vi "pulse_generator_multiheater_partial_refnum.vi"(2 "Stop! Refnum":refnum<vi>, 3 "Pulse Generator Control Multiheater Refnums":T1) -> ()   [LabVIEW 2017]
uses:
  pulse_generator_controls_multiheater_refnums.ctl
  <vilib>/Utility/error.llb/DialogType.ctl
  <vilib>/DAQmx/write.llb/DAQmx Write (Digital 1D Bool NChan 1Samp 1Line).vi
  <vilib>/DAQmx/write.llb/DAQmx Write (Digital Wfm 1Chan NSamp).vi
  <vilib>/DAQmx/write.llb/DAQmx Write (Counter 1D Frequency 1Chan NSamp).vi
  <vilib>/DAQmx/read.llb/DAQmx Read (Counter DBL 1Chan 1Samp).vi
  <vilib>/DAQmx/create/channels.llb/DAQmx Create Channel (CI-Position-Angular Encoder).vi
  <vilib>/DAQmx/create/channels.llb/DAQmx Create Channel (DO-Digital Output).vi
  <vilib>/DAQmx/configure/timing.llb/DAQmx Timing (Sample Clock).vi
  <vilib>/DAQmx/create/channels.llb/DAQmx Create Channel (CO-Pulse Generation-Frequency).vi
  <vilib>/DAQmx/configure/timing.llb/DAQmx Timing (Implicit).vi
  <vilib>/DAQmx/configure/trigger.llb/DAQmx Start Trigger (Digital Edge).vi
  <vilib>/Waveform/DWDTOps.llb/DWDT Uncompress Digital.vi
  <vilib>/DAQmx/miscellaneous.llb/DAQmx Fill In Error Info.vi
panel:
  out "data":dbl format="%0.2f"
  out "Stopped!":bool caption="OK"
  in  "Stop! Local":bool
  out "message":string=" INSTRUCTIONS:\r\rNormal Use:  When using subVIs that incorporate the error in/error out (or error I/O) structure, place this handler where you want to inform the user of an error, typically at the end of the I/O data path, as the last action of the program.  If the error in error? is ERROR, the handler creates a message describing the error and its source.  If the type of dialog = 1 (default), the message is displayed to the user, who can only acknowedge it.  If the type = 2, the user can acknowledge the message or abort execution; aborting a program with active I/O is not recommended.  If the type = 0, no message is displayed; this is used to process the error programmatically, and the error out cluster elements are wired to individual terminals for that reason.  \r\rOther Use:\n\r\nlocal testing.  To test the error code of a subVI or function that does not have the error I/O structure, you can wire its error code and a source string to the local error code and error source inputs.  If error in error? indicates no error and error code is not equal to 0, the local code and source are substituted for the error in values, and error? is set TRUE (ERROR)."
  in  "SwitchHelper":bool
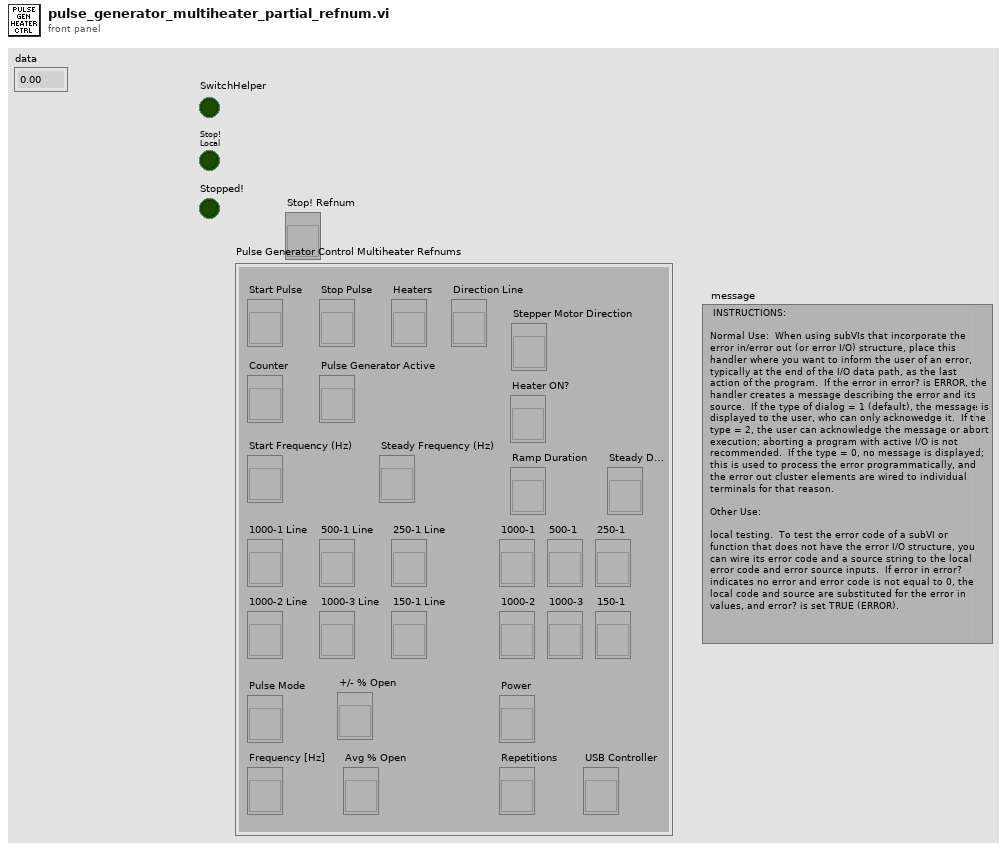
[diagram p1: front panel]
types:
  T1 = typedef "pulse_generator_controls_multiheater_refnums.ctl" = cluster{"Start Pulse":refnum<vi>, "Stop Pulse":refnum<vi>, "Heaters":refnum<vi>, "Counter":refnum<vi>, "Start Frequency (Hz)":refnum<vi>, "Pulse Generator Active":refnum<vi>, "Stepper Motor Direction":refnum<vi>, "Ramp Duration":refnum<vi>, "Direction Line":refnum<vi>, "1000-1 Line":refnum<vi>, "1000-2 Line":refnum<vi>, "1000-3 Line":refnum<vi>, "500-1 Line":refnum<vi>, "250-1 Line":refnum<vi>, "1000-1":refnum<vi>, "1000-2":refnum<vi>, "1000-3":refnum<vi>, "500-1":refnum<vi>, "250-1":refnum<vi>, "150-1":refnum<vi>, "Heater ON?":refnum<vi>, "150-1 Line":refnum<vi>, "Power":refnum<vi>, "Steady Frequency (Hz)":refnum<vi>, "Steady Duration ":refnum<vi>, "Pulse Mode":refnum<vi>, "Frequency [Hz]":refnum<vi>, "Avg % Open":refnum<vi>, "Repetitions":refnum<vi>, "+/- % Open":refnum<vi>, "USB Controller":refnum<vi>}
  T2 = enum8{"Enabled", "Disabled", "Disabled and Grayed Out"}
  T3 = typedef "DialogType.ctl" = u16
  T4 = cluster{"1000-1":refnum<vi>, "1000-2":refnum<vi>, "1000-3":refnum<vi>, "500-1":refnum<vi>, "250-1":refnum<vi>, "150-1":refnum<vi>}
  T5 = cluster{"1000-1 Line":refnum<vi>, "1000-2 Line":refnum<vi>, "1000-3 Line":refnum<vi>, "500-1 Line":refnum<vi>, "250-1 Line":refnum<vi>, "150-1 Line":refnum<vi>}
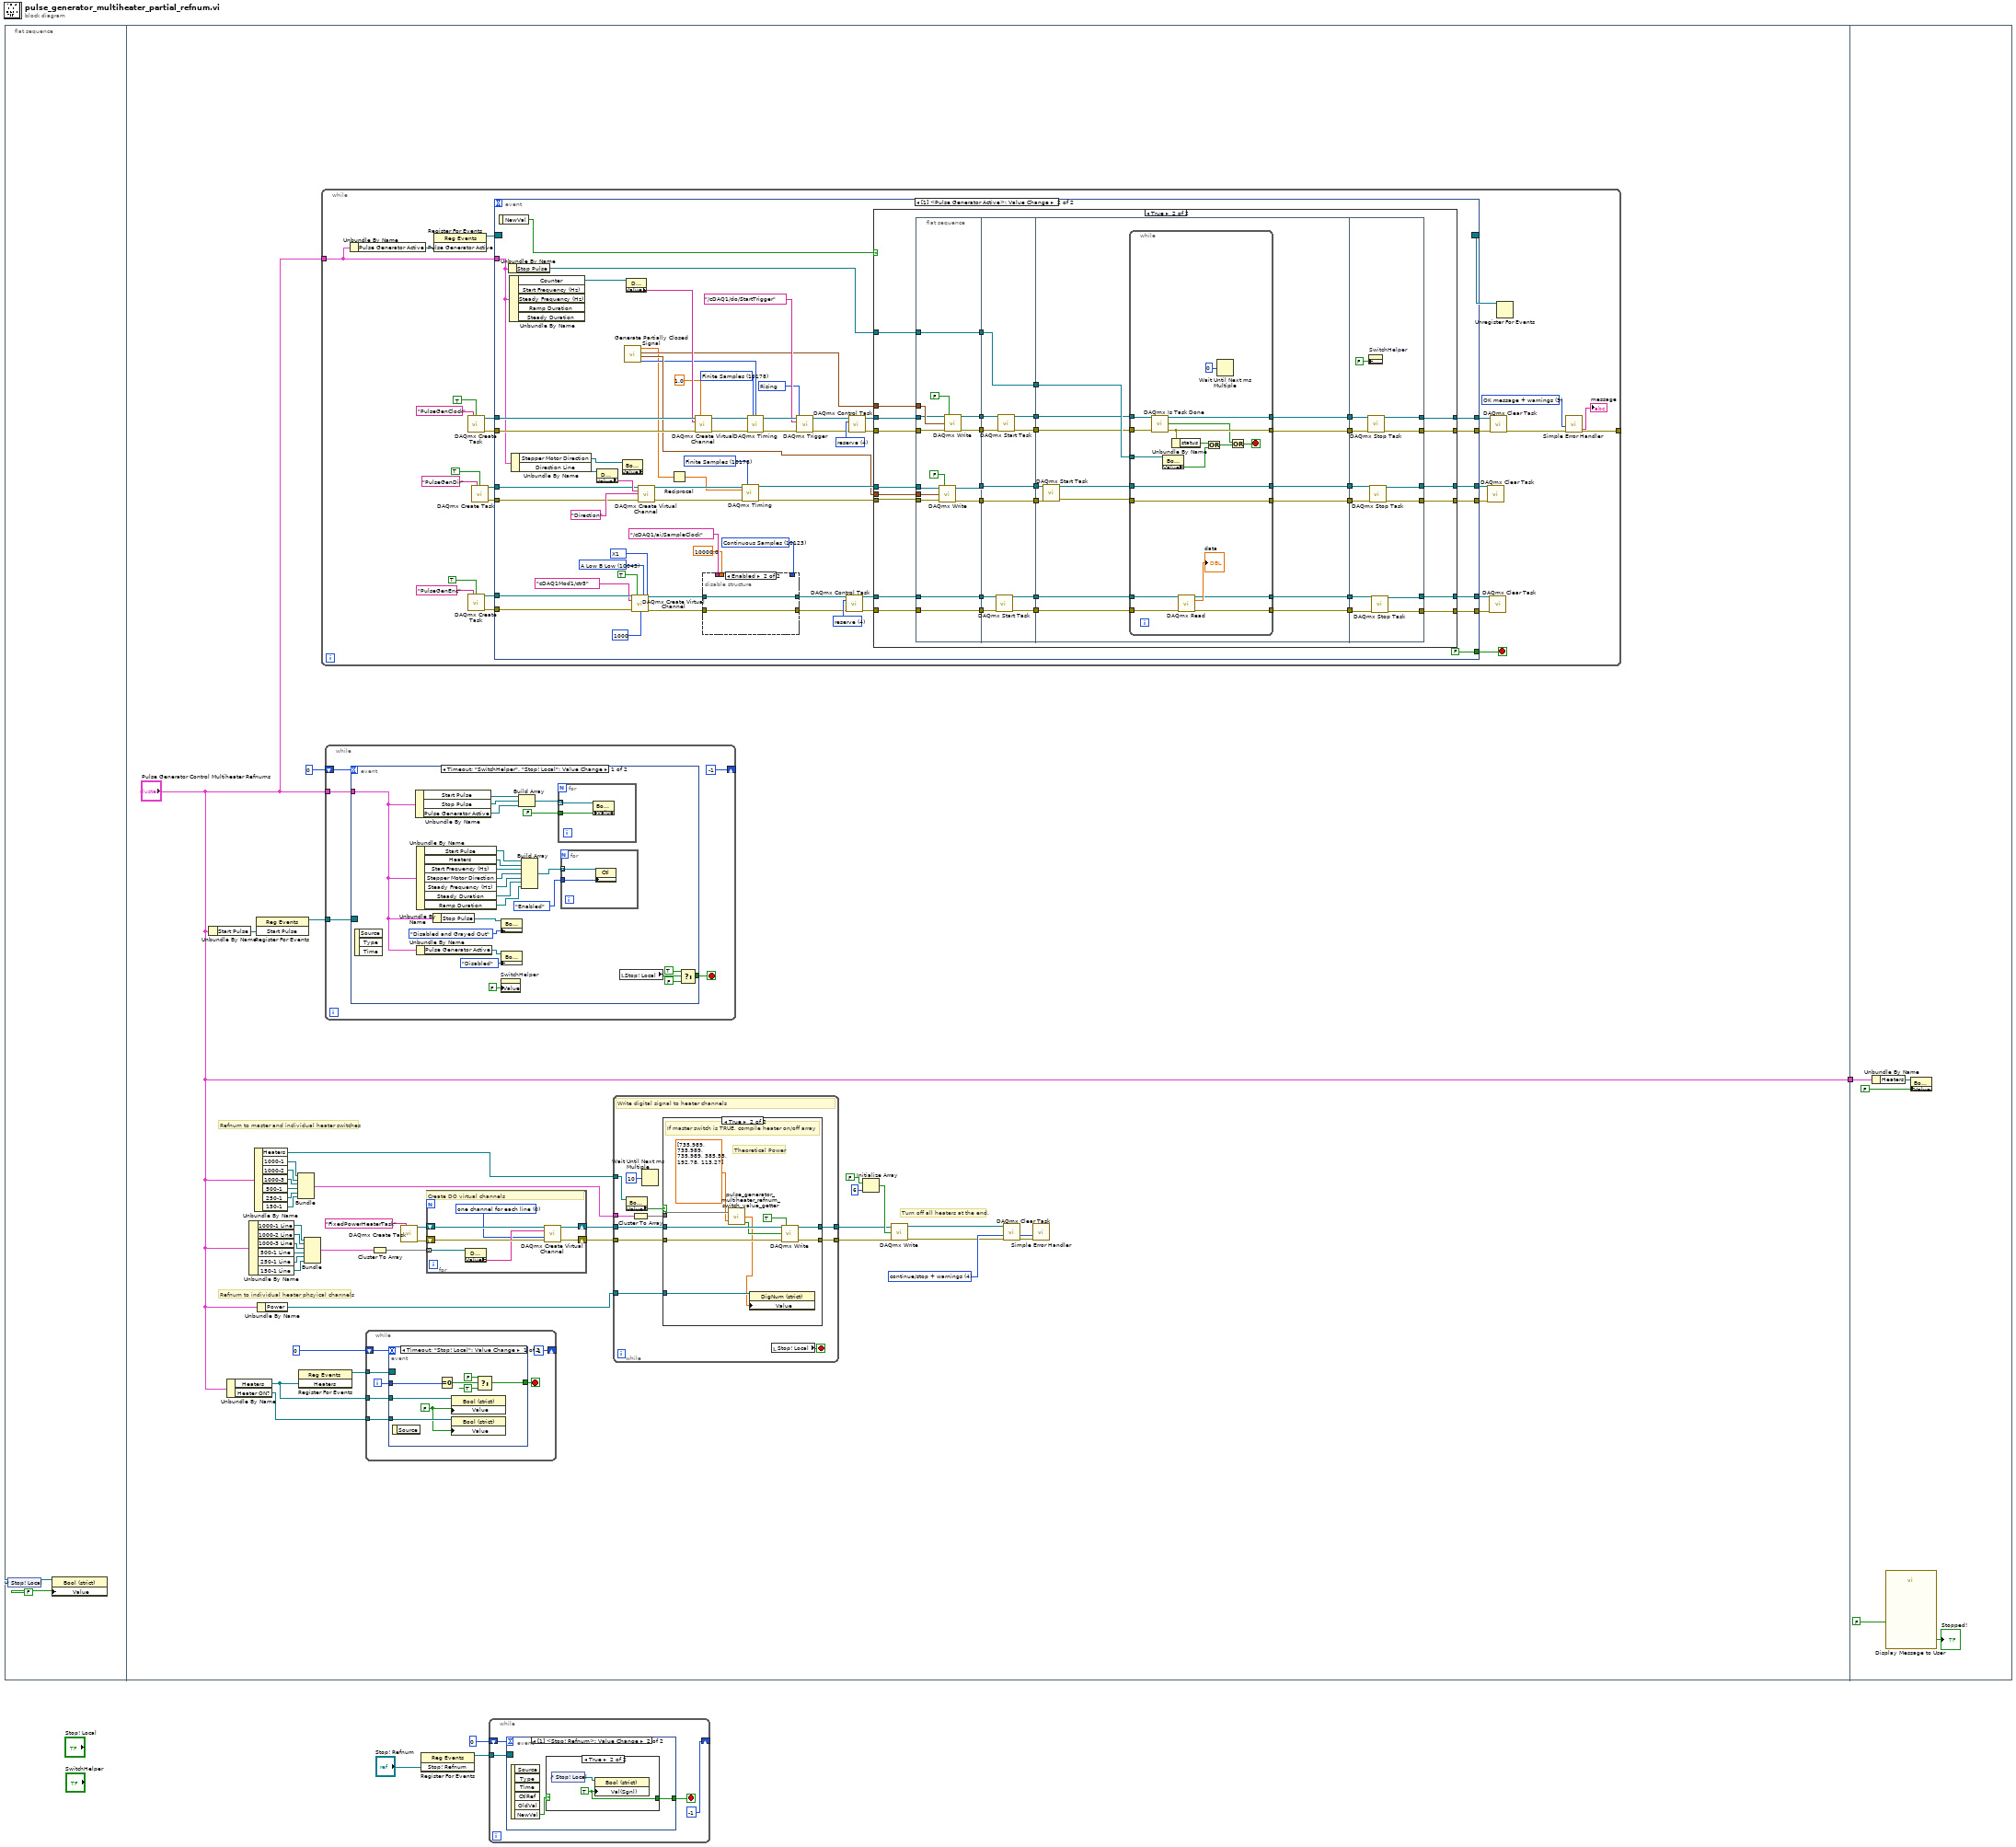
[diagram p0: block diagram]
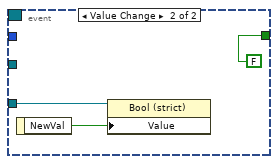
[diagram p2: hidden frame]
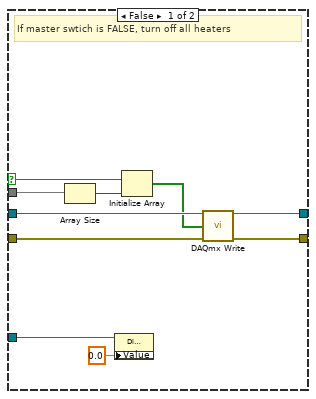
[diagram p3: hidden frame]
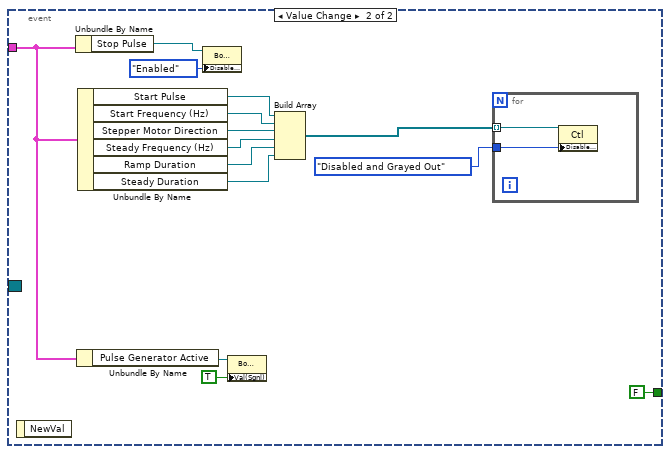
[diagram p4: hidden frame]
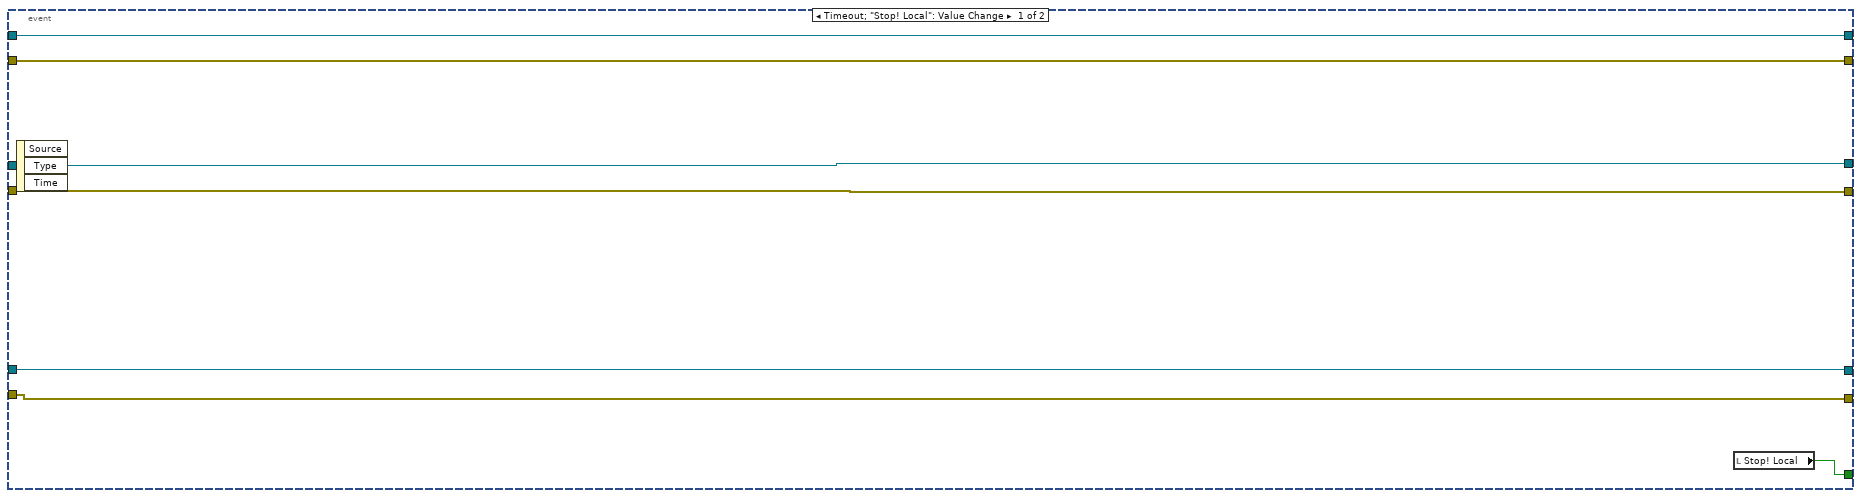
[diagram p5: hidden frame]
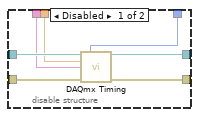
[diagram p6: hidden frame]
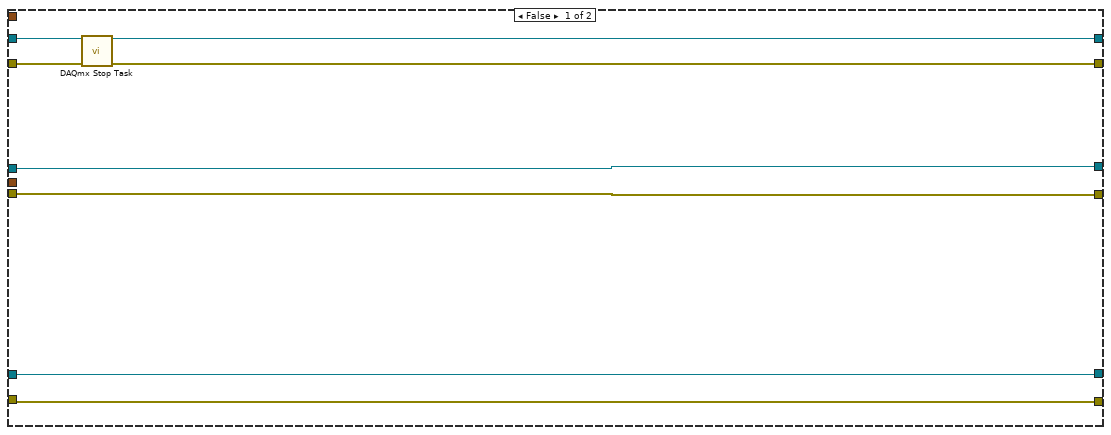
[diagram p7: hidden frame]
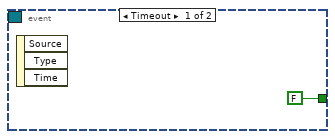
[diagram p8: hidden frame]
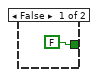
[diagram p9: hidden frame]
diagram:
  n1 = flat-sequence {
    tunnel: ["Pulse Generator Control Multiheater Refnums"] -> w1
    tunnel: w1 -> [w371]
    frame #0 {
      n2 = control-ref of="Stop! Local"() -> (w5:refnum<vi>)
      n3 = property class="Bool (strict)"(reference=w5, "Value"=FALSE) -> ()  [unwired: 1 in, 2 out]
    }
    frame #1 {
      w40 = T3 4 items=["no dialog", "OK message", "continue or stop message", "OK message + warnings", "continue/stop + warnings"] ("type of dialog (OK msg:1)")
      # "Turn off all heaters at the end."
      # "Refnum to individual heater phsyical channels"
      # "Refnum to master and individual heater switches"
      n4 = Unbundle By Name("Pulse Generator Control Multiheater Refnums") -> ("Start Pulse"=w43:refnum<vi>)
      n5 = Unbundle By Name("Pulse Generator Control Multiheater Refnums") -> ("Heaters"=w35:refnum<vi>, "Heater ON?"=w17:refnum<vi>)
      n6 = Unbundle By Name("Pulse Generator Control Multiheater Refnums") -> ("1000-1 Line"=w14:refnum<vi>, "1000-2 Line"=w13:refnum<vi>, "1000-3 Line"=w12:refnum<vi>, "500-1 Line"=w11:refnum<vi>, "250-1 Line"=w10:refnum<vi>, "150-1 Line"=w9:refnum<vi>)
      n7 = Unbundle By Name("Pulse Generator Control Multiheater Refnums") -> ("Heaters"=w34:refnum<vi>, "1000-1"=w33:refnum<vi>, "1000-2"=w32:refnum<vi>, "1000-3"=w31:refnum<vi>, "500-1"=w30:refnum<vi>, "250-1"=w28:refnum<vi>, "150-1"=w18:refnum<vi>)
      n8 = register-events(w43) -> (reference out=w44:refnum<event-registration>)  [unwired: 2 in, 1 out]
      n9 = Unbundle By Name("Pulse Generator Control Multiheater Refnums") -> ("Power"=w7:refnum<vi>)
      n10 = Bundle("1000-1"=w33, "1000-2"=w32, "1000-3"=w31, "500-1"=w30, "250-1"=w28, "150-1"=w18) -> (w15:T4)  [unwired: 1 in]
      n11 = register-events(w35) -> (reference out=w39:refnum<event-registration>)  [unwired: 2 in, 1 out]
      n12 = Bundle("1000-1 Line"=w14, "1000-2 Line"=w13, "1000-3 Line"=w12, "500-1 Line"=w11, "250-1 Line"=w10, "150-1 Line"=w9) -> (w16:T5)  [unwired: 1 in]
      n13 = while {
        tunnel: [w162] -> _
        tunnel: "Pulse Generator Control Multiheater Refnums" -> [w161]
        stop <- w170 stop-if-true
        w173 = T3 3 items=["no dialog", "OK message", "continue or stop message", "OK message + warnings", "continue/stop + warnings"] ("type of dialog (OK msg:1)")
        n14 = Unbundle By Name(w161) -> ("Pulse Generator Active"=w163:refnum<vi>)
        n15 = register-events(w163) -> (reference out=w175:refnum<event-registration>)  [unwired: 2 in, 1 out]
        n16 = call <vilib>:"DAQmx Create Task.vi"("new task name"="PulseGenClock", "auto cleanup"=TRUE) -> ("task out"=w172:refnum<k21>, "error out"=w171:errorcluster)  [unwired: 12 in]
        n17 = call <vilib>:"DAQmx Create Task.vi"("new task name"="PulseGenEnc", "auto cleanup"=TRUE) -> ("task out"=w154:refnum<k21>, "error out"=w153:errorcluster)  [unwired: 12 in]
        n18 = call <vilib>:"DAQmx Create Task.vi"("new task name"="PulseGenDir", "auto cleanup"=TRUE) -> ("task out"=w168:refnum<k21>, "error out"=w167:errorcluster)  [unwired: 12 in]
        n19 = event shown="[1] <Pulse Generator Active>: Value Change" {
          selector: w175 -> [_ _]
          dyn-events: [_ _] -> w160
          timeout: _ -> [_ _]
          tunnel: [w183 w224] -> w177
          tunnel: [w184 w223] -> w176
          tunnel: w172 -> [w184 w242]
          tunnel: w171 -> [w183 w241]
          tunnel: [w182 FALSE ("Stop! Local")] -> w170
          tunnel: w168 -> [w181 w238]
          tunnel: w167 -> [w180 w237]
          tunnel: [w181 w227] -> w158
          tunnel: [w180 w226] -> w157
          tunnel: w161 -> [_ w228]
          tunnel: w154 -> [w179 w212]
          tunnel: w153 -> [w178 w213]
          tunnel: [w179 w191] -> w151
          tunnel: [w178 w192] -> w152
          event Timeout; "Stop! Local": Value Change {
            n20 = event-data() -> ()  [unwired: 1 in, 3 out]
            n21 = local read "Stop! Local"() -> (w182:bool)
          }
          event Value Change {
            w185 = 10123 items=["Finite Samples"=10178, "Continuous Samples"=10123, "Hardware Timed Single Point"=12522] ("sample mode")
            w195 = 10178 items=["Finite Samples"=10178, "Continuous Samples"=10123, "Hardware Timed Single Point"=12522] ("sample mode")
            w206 = 10090 items=["X1"=10090, "X2"=10091, "X4"=10092, "Two Pulse Counting"=10313] ("decoding type")
            w207 = 4 items=["verify"=2, "reserve"=4, "commit"=3, "unreserve"=5, "abort"=6] ("action")
            w209 = 10043 items=["A High B High"=10040, "A High B Low"=10041, "A Low B High"=10042, "A Low B Low"=10043] ("z index phase")
            w215 = 10280 items=["Rising"=10280, "Falling"=10171] ("edge")
            w222 = 4 items=["verify"=2, "reserve"=4, "commit"=3, "unreserve"=5, "abort"=6] ("action")
            w243 = 10178 items=["Finite Samples"=10178, "Continuous Samples"=10123, "Hardware Timed Single Point"=12522] ("sample mode")
            n22 = event-data() -> ("NewVal"=w244:bool)  [unwired: 1 in]
            n23 = Unbundle By Name(w228) -> ("Stop Pulse"=w231:refnum<vi>)
            n24 = Unbundle By Name(w228) -> ("Counter"=w230:refnum<vi>)  [unwired: 4 out]
            n25 = Unbundle By Name(w228) -> ("Stepper Motor Direction"=w221:refnum<vi>, "Direction Line"=w232:refnum<vi>)
            n26 = property class="DAQmxName"(reference=w232) -> ("Value"=w240:string)  [unwired: 1 in, 2 out]
            n27 = property class="Bool (strict)" props=["Value"](reference=w221) -> ()  [unwired: 1 in, 3 out]
            n28 = call "Generate Partially Closed Signal.vi"() -> ("Total # of Frequency Samples"=w188:i32, "Digital Waveform Graph"=w189:digitalwaveform, "CO Frequency"=w190:cluster{"duty cycle":dbl, "frequency":dbl}[], "dt"=w186:dbl)  [unwired: 6 in, 1 out]
            n29 = property class="DAQmxName"(reference=w230) -> ("Value"=w229:string)  [unwired: 1 in, 2 out]
            n30 = call-poly <vilib>:"DAQmx Create Virtual Channel.vi"("task in"=w212, "z index enable"=TRUE, "z index phase"=w209, "counter"=tag "cDAQ1Mod1/ctr3", "decoding type"=w206, "error in"=w213, "pulses per revolution"=u32 1000) -> ("task out"=w199:refnum<k21>, "error out"=w198:errorcluster)  [unwired: 7 in]
            n31 = call-poly <vilib>:"DAQmx Create Virtual Channel.vi"("task in"=w238, "lines"=w240, "name to assign"="Direction", "error in"=w237) -> ("task out"=w203:refnum<k21>, "error out"=w202:errorcluster)  [unwired: 10 in]
            n32 = Reciprocal(x=w186) -> (1/x=w187:dbl)
            n33 = call-poly <vilib>:"DAQmx Create Virtual Channel.vi"("task in"=w242, "frequency"=1.0, "counter"=w229, "error in"=w241) -> ("task out"=w236:refnum<k21>, "error out"=w235:errorcluster)  [unwired: 10 in]
            n34 = disable-structure shown="Enabled" {
              disable-tunnel: w199 -> [w251 w253]
              disable-tunnel: w198 -> [w250 w252]
              disable-tunnel: [w249 w252] -> w197
              disable-tunnel: [w248 w253] -> w196
              disable-tunnel: w185 -> [w247 _]
              disable-tunnel: tag "/cDAQ1/ai/SampleClock" ("source") -> [w246 _]
              disable-tunnel: 10000.0 ("rate") -> [w245 _]
              frame Disabled {
                n35 = call-poly <vilib>:"DAQmx Timing.vi"("task/channels in"=w251, "sample mode"=w247, "rate"=w245, "source"=w246, "error in"=w250) -> ("task out"=w248:refnum<k21>, "error out"=w249:errorcluster)  [unwired: 9 in]
              }
              frame Enabled {
              }
            }
            n36 = call-poly <vilib>:"DAQmx Timing.vi"("task/channels in"=w203, "sample mode"=w195, "rate"=w187, "error in"=w202) -> ("task out"=w201:refnum<k21>, "error out"=w200:errorcluster)  [unwired: 10 in]
            n37 = call-poly <vilib>:"DAQmx Timing.vi"("task/channels in"=w236, "sample mode"=w243, "samples per channel"=w188, "error in"=w235) -> ("task out"=w220:refnum<k21>, "error out"=w219:errorcluster)  [unwired: 10 in]
            n38 = call-poly <vilib>:"DAQmx Trigger.vi"("task/channels in"=w220, "source"=tag "/cDAQ1/do/StartTrigger" ("Start.DigEdge.Src"), "edge"=w215, "error in"=w219) -> ("task out"=w218:refnum<k21>, "error out"=w217:errorcluster)  [unwired: 10 in]
            n39 = call <vilib>:"DAQmx Control Task.vi"("task/channels in"=w196, "action"=w207, "error in"=w197) -> ("task out"=w205:refnum<k21>, "error out"=w204:errorcluster)  [unwired: 11 in]
            n40 = call <vilib>:"DAQmx Control Task.vi"("task/channels in"=w218, "action"=w222, "error in"=w217) -> ("task out"=w233:refnum<k21>, "error out"=w234:errorcluster)  [unwired: 11 in]
            n41 = case shown="True" w244 {
              tunnel: w233 -> [w261 w294]
              tunnel: w234 -> [w260 w285]
              tunnel: [w258 w296] -> w223
              tunnel: [w259 w295] -> w224
              tunnel: w231 -> [_ w292]
              tunnel: w201 -> [w257 w291]
              tunnel: w200 -> [w256 w284]
              tunnel: [w257 w290] -> w227
              tunnel: [w256 w288] -> w226
              tunnel: w190 -> [_ w283]
              tunnel: w189 -> [_ w272]
              tunnel: w205 -> [w255 w271]
              tunnel: w204 -> [w254 w270]
              tunnel: [w255 w262] -> w191
              tunnel: [w254 w263] -> w192
              frame False {
                n42 = call <vilib>:"DAQmx Stop Task.vi"("task/channels in"=w261, "error in"=w260) -> ("task out"=w258:refnum<k21>, "error out"=w259:errorcluster)  [unwired: 12 in]
              }
              frame True {
                n43 = flat-sequence {
                  tunnel: w291 -> [w310]
                  tunnel: w292 -> [w311]
                  tunnel: w294 -> [w304]
                  tunnel: w285 -> [w303]
                  tunnel: [w311] -> w282
                  tunnel: [w307] -> w280
                  tunnel: [w308] -> w279
                  tunnel: w284 -> [w309]
                  tunnel: w283 -> [w305]
                  tunnel: [w302] -> w277
                  tunnel: [w301] -> w276
                  tunnel: w272 -> [w299]
                  tunnel: w271 -> [w298]
                  tunnel: w270 -> [w297]
                  tunnel: [w298] -> w269
                  tunnel: [w297] -> w268
                  tunnel: w282 -> [w322]
                  tunnel: [w322] -> w281
                  tunnel: w280 -> [w316]
                  tunnel: w279 -> [w317]
                  tunnel: [w317] -> w278
                  tunnel: w277 -> [w321]
                  tunnel: w276 -> [w320]
                  tunnel: [w318] -> w275
                  tunnel: [w316] -> w274
                  tunnel: [w319] -> w273
                  tunnel: w269 -> [w315]
                  tunnel: w268 -> [w314]
                  tunnel: [w313] -> w267
                  tunnel: [w312] -> w266
                  tunnel: [w337] -> w293
                  tunnel: [w331] -> w289
                  tunnel: w281 -> [w335]
                  tunnel: [w332] -> w287
                  tunnel: [w336] -> w286
                  tunnel: w278 -> [w326]
                  tunnel: w275 -> [w333]
                  tunnel: w274 -> [w325]
                  tunnel: w273 -> [w334]
                  tunnel: w267 -> [w330]
                  tunnel: w266 -> [w329]
                  tunnel: [w328] -> w265
                  tunnel: [w327] -> w264
                  tunnel: [w365] -> w295
                  tunnel: [w366] -> w296
                  tunnel: w293 -> [w367]
                  tunnel: [w361] -> w290
                  tunnel: w289 -> [w362]
                  tunnel: [w360] -> w288
                  tunnel: w287 -> [w363]
                  tunnel: w286 -> [w364]
                  tunnel: w265 -> [w357]
                  tunnel: w264 -> [w356]
                  tunnel: [w358] -> w262
                  tunnel: [w359] -> w263
                  frame #0 {
                    n44 = call-poly <vilib>:"DAQmx Write.vi"("task/channels in"=w310, "auto start"=FALSE, "data"=w299, "error in"=w309) -> ("task out"=w308:refnum<k21>, "error out"=w307:errorcluster)  [unwired: 9 in, 1 out]
                    n45 = call-poly <vilib>:"DAQmx Write.vi"("task/channels in"=w304, "auto start"=FALSE, "data"=w305, "error in"=w303) -> ("task out"=w302:refnum<k21>, "error out"=w301:errorcluster)  [unwired: 9 in, 1 out]
                  }
                  frame #1 {
                    n46 = call <vilib>:"DAQmx Start Task.vi"("task/channels in"=w315, "error in"=w314) -> ("task out"=w313:refnum<k21>, "error out"=w312:errorcluster)  [unwired: 12 in]
                    n47 = call <vilib>:"DAQmx Start Task.vi"("task/channels in"=w321, "error in"=w320) -> ("task out"=w318:refnum<k21>, "error out"=w319:errorcluster)  [unwired: 12 in]
                  }
                  frame #2 {
                    n48 = call <vilib>:"DAQmx Start Task.vi"("task/channels in"=w326, "error in"=w325) -> ("task out"=w323:refnum<k21>, "error out"=w324:errorcluster)  [unwired: 12 in]
                    n49 = while {
                      tunnel: w334 -> [w354]
                      tunnel: w333 -> [w355]
                      tunnel: [w345] -> w337
                      tunnel: [w351] -> w336
                      tunnel: w335 -> [w347]
                      tunnel: w323 -> [w344]
                      tunnel: w324 -> [w343]
                      tunnel: [w344] -> w332
                      tunnel: [w343] -> w331
                      tunnel: w330 -> [w342]
                      tunnel: w329 -> [w341]
                      tunnel: [w339] -> w328
                      tunnel: [w338] -> w327
                      stop <- w349 stop-if-true
                      n50 = call <vilib>:"DAQmx Is Task Done.vi"("task/channels in"=w355, "error in"=w354) -> ("task out"=w345:refnum<k21>, "task done?"=w348:bool, "error out"=w351:errorcluster)  [unwired: 11 in]
                      n51 = property class="Bool (strict)"(reference=w347) -> ("Value"=w346:bool)  [unwired: 1 in, 2 out]
                      n52 = Unbundle By Name(w351) -> ("status"=w352:bool)
                      n53 = call-poly <vilib>:"DAQmx Read.vi"("task/channels in"=w342, "error in"=w341) -> ("task out"=w339:refnum<k21>, "data"=→"data":dbl, "error out"=w338:errorcluster)  [unwired: 11 in]
                      n54 = Or(x=w352, y=w346) -> (x .or. y?=w350:bool)
                      n55 = Wait Until Next ms Multiple(millisecond multiple=u32 0) -> ()  [unwired: 1 out]
                      n56 = Or(x=w348, y=w350) -> (x .or. y?=w349:bool)
                    }
                  }
                  frame #3 {
                    n57 = call <vilib>:"DAQmx Stop Task.vi"("task/channels in"=w367, "error in"=w364) -> ("task out"=w366:refnum<k21>, "error out"=w365:errorcluster)  [unwired: 12 in]
                    n58 = property on="SwitchHelper" class="Bool (strict)"("Val(Sgnl)"=FALSE ("Value (Signaling)")) -> ()  [unwired: 2 in, 2 out]
                    n59 = call <vilib>:"DAQmx Stop Task.vi"("task/channels in"=w363, "error in"=w362) -> ("task out"=w361:refnum<k21>, "error out"=w360:errorcluster)  [unwired: 12 in]
                    n60 = call <vilib>:"DAQmx Stop Task.vi"("task/channels in"=w357, "error in"=w356) -> ("task out"=w358:refnum<k21>, "error out"=w359:errorcluster)  [unwired: 12 in]
                  }
                }
              }
            }
          }
        }
        n61 = call <vilib>:"DAQmx Clear Task.vi"("task in"=w158, "error in"=w157) -> ()  [unwired: 13 in, 1 out]
        n62 = call <vilib>:"DAQmx Clear Task.vi"("task in"=w151, "error in"=w152) -> ()  [unwired: 13 in, 1 out]
        n63 = call <vilib>:"DAQmx Clear Task.vi"("task in"=w176, "error in"=w177) -> ("error out"=w159:errorcluster)  [unwired: 13 in]
        n64 = Unregister For Events(event registration refnum=w160) -> ()  [unwired: 1 in, 1 out]
        n65 = call <vilib>:"Simple Error Handler.vi"("type of dialog (OK msg:1)"=w173, "error in (no error)"=w159) -> ("error out"=w162:errorcluster, "message"=→"message":string)  [unwired: 3 in, 3 out]
      }
      n66 = while {
        shift-right: [-1] -> _
        shift-left: 0 -> [w106]
        tunnel: w44 -> [w104]
        tunnel: "Pulse Generator Control Multiheater Refnums" -> [w102]
        stop <- w103 stop-if-true
        n67 = event shown="[0] Timeout;  \"SwitchHelper\", \"Stop! Local\": Value Change" {
          selector: w104 -> [_ _]
          dyn-events: _ -> [_ _]
          timeout: w106 -> [_ _]
          tunnel: [w127 FALSE ("Value")] -> w103
          tunnel: w102 -> [w109 w137]
          event Timeout; "SwitchHelper", "Stop! Local": Value Change {
            n68 = event-data() -> ()  [unwired: 1 in, 3 out]
            n69 = Unbundle By Name(w109) -> ("Start Pulse"=w116:refnum<vi>, "Stop Pulse"=w115:refnum<vi>, "Pulse Generator Active"=w114:refnum<vi>)
            n70 = Unbundle By Name(w109) -> ("Start Pulse"=w120:refnum<vi>, "Heaters"=w124:refnum<vi>, "Start Frequency (Hz)"=w123:refnum<vi>, "Stepper Motor Direction"=w122:refnum<vi>, "Steady Frequency (Hz)"=w121:refnum<vi>, "Steady Duration"=w108:refnum<vi>, "Ramp Duration"=w107:refnum<vi>)
            n71 = Unbundle By Name(w109) -> ("Pulse Generator Active"=w112:refnum<vi>)
            n72 = Unbundle By Name(w109) -> ("Stop Pulse"=w111:refnum<vi>)
            n73 = property on="SwitchHelper" class="Bool (strict)"("Value"=FALSE) -> ()  [unwired: 2 in, 2 out]
            n74 = property class="Bool (strict)"(reference=w111, "DisabledEnum"=T2."Disabled and Grayed Out" ("Disabled")) -> ()  [unwired: 1 in, 2 out]
            n75 = property class="Bool (strict)"(reference=w112, "DisabledEnum"=T2."Disabled" ("Disabled")) -> ()  [unwired: 1 in, 2 out]
            n76 = Build Array(w116, w115, w114) -> (w117:refnum<vi>[])
            n77 = Build Array(w120, w124, w123, w122, w121, w108, w107) -> (w119:refnum<vi>[])
            n78 = for {
              tunnel: w117 -> [w132] mode=indexing
              tunnel: FALSE ("Value") -> [w131]
              n79 = property class="Bool (strict)"(reference=w132, "Value"=w131) -> ()  [unwired: 1 in, 2 out]
            }
            n80 = for {
              tunnel: w119 -> [w134] mode=indexing
              tunnel: T2."Enabled" ("Disabled") -> [w133]
              n81 = property class="Ctl"(reference=w134, "DisabledEnum"=w133) -> ()  [unwired: 1 in, 2 out]
            }
            n82 = local read "Stop! Local"() -> (w128:bool)
            n83 = Select(t=TRUE ("Value"), s=w128, f=FALSE ("Value")) -> (s? t:f=w127:bool)
          }
          event Value Change {
            n84 = event-data() -> ()  [unwired: 1 in, 1 out]
            n85 = Unbundle By Name(w137) -> ("Stop Pulse"=w141:refnum<vi>)
            n86 = Unbundle By Name(w137) -> ("Pulse Generator Active"=w139:refnum<vi>)
            n87 = Unbundle By Name(w137) -> ("Start Pulse"=w144:refnum<vi>, "Start Frequency (Hz)"=w145:refnum<vi>, "Stepper Motor Direction"=w146:refnum<vi>, "Steady Frequency (Hz)"=w147:refnum<vi>, "Ramp Duration"=w136:refnum<vi>, "Steady Duration"=w135:refnum<vi>)
            n88 = property class="Bool (strict)"(reference=w141, "DisabledEnum"=T2."Enabled" ("Disabled")) -> ()  [unwired: 1 in, 2 out]
            n89 = property class="Bool (strict)"(reference=w139, "Val(Sgnl)"=TRUE ("Value")) -> ()  [unwired: 1 in, 2 out]
            n90 = Build Array(w144, w145, w146, w147, w136, w135) -> (w143:refnum<vi>[])
            n91 = for {
              tunnel: w143 -> [w150] mode=indexing
              tunnel: T2."Disabled and Grayed Out" ("Disabled") -> [w149]
              n92 = property class="Ctl"(reference=w150, "DisabledEnum"=w149) -> ()  [unwired: 1 in, 2 out]
            }
          }
        }
      }
      n93 = while {
        tunnel: w39 -> [w59]
        shift-right: [-1 ("millisecond multiple")] -> _
        shift-left: 0 ("millisecond multiple") -> [w58]
        tunnel: w35 -> [w56]
        tunnel: w17 -> [w53]
        i -> [w55]
        stop <- w54 stop-if-true
        n94 = event shown="[0] Timeout;  \"Stop! Local\": Value Change" {
          selector: w59 -> [_ _]
          dyn-events: _ -> [_ _]
          timeout: w58 -> [_ _]
          tunnel: w56 -> [w67 _]
          tunnel: w55 -> [w65 _]
          tunnel: [w62 FALSE ("f")] -> w54
          tunnel: w53 -> [w61 w68]
          event Timeout; "Stop! Local": Value Change {
            w60 = FALSE ("Value")
            n95 = event-data() -> ()  [unwired: 1 in, 1 out]
            n96 = Equal To 0?(x=w65) -> (x = 0?=w66:bool)
            n97 = property class="Bool (strict)"(reference=w67, "Value"=w60) -> ()  [unwired: 1 in, 2 out]
            n98 = property class="Bool (strict)"(reference=w61, "Value"=w60) -> ()  [unwired: 1 in, 2 out]
            n99 = Select(t=FALSE, s=w66, f=TRUE) -> (s? t:f=w62:bool)
          }
          event Value Change {
            n100 = event-data() -> ("NewVal"=w69:bool)  [unwired: 1 in]
            n101 = property class="Bool (strict)"(reference=w68, "Value"=w69) -> ()  [unwired: 1 in, 2 out]
          }
        }
      }
      n102 = Cluster To Array(cluster=w16) -> (array=w29:refnum<vi>[])
      n103 = call <vilib>:"DAQmx Create Task.vi"("new task name"="FixedPowerHeaterTask") -> ("task out"=w38:refnum<k21>, "error out"=w37:errorcluster)  [unwired: 13 in]
      n104 = for {
        tunnel: w29 -> [w48] mode=indexing
        shift-right: [w52] -> w21
        shift-left: w38 -> [w50]
        shift-right: [w51] -> w20
        shift-left: w37 -> [w49]
        w46 = 0 items=["one channel for each line", "one channel for all lines"] ("line grouping")
        # "Create DO virtual channels"
        n105 = property class="DAQmxName"(reference=w48) -> ("Value"=w47:string)  [unwired: 1 in, 2 out]
        n106 = call-poly <vilib>:"DAQmx Create Virtual Channel.vi"("task in"=w50, "lines"=w47, "line grouping"=w46, "error in"=w49) -> ("task out"=w52:refnum<k21>, "error out"=w51:errorcluster)  [unwired: 10 in]
      }
      n107 = while {
        tunnel: w21 -> [w79]
        tunnel: w20 -> [w78]
        tunnel: w34 -> [w75]
        tunnel: [w77] -> w23
        tunnel: [w76] -> w22
        tunnel: w15 -> [w73]
        tunnel: w7 -> [w71]
        stop <- w80 stop-if-true
        # "Write digital signal to heater channels"
        n108 = property class="Bool (strict)"(reference=w75) -> ("Value"=w74:bool)  [unwired: 1 in, 2 out]
        n109 = Cluster To Array(cluster=w73) -> (array=w72:refnum<vi>[])
        n110 = Wait Until Next ms Multiple(millisecond multiple=u32 10) -> ()  [unwired: 1 out]
        n111 = case shown="True" w74 {
          selector: w74 -> [w84 _]
          tunnel: w79 -> [w91 w100]
          tunnel: w78 -> [w90 w99]
          tunnel: [w88 w101] -> w77
          tunnel: [w89 w98] -> w76
          tunnel: w72 -> [w86 w96]
          tunnel: w71 -> [w83 w93]
          frame False {
            # "If master swtich is FALSE, turn off all heaters"
            n112 = Array Size(array=w86) -> (size(s)=w87:i32)
            n113 = property class="DigNum (strict)"(reference=w83, "Value"=0.0) -> ()  [unwired: 1 in, 2 out]
            n114 = Initialize Array(w84, w87) -> (w85:bool[])
            n115 = call-poly <vilib>:"DAQmx Write.vi"("task/channels in"=w91, "data"=w85, "error in"=w90) -> ("task out"=w88:refnum<k21>, "error out"=w89:errorcluster)  [unwired: 10 in, 1 out]
          }
          frame True {
            # "Theoretical Power"
            # "If master switch is TRUE, compile heater on/off array"
            n116 = call "pulse_generator_multiheater_refnum_switch_value_getter.vi"("On/Off Refnums"=w96, "Power Array"=dbl[] [735.989, 735.989, 735.989, 385.55, 192.78, 113.27]) -> ("Total Power"=w92:dbl, "Digital"=w95:bool[])  [unwired: 1 out]
            n117 = property class="DigNum (strict)"(reference=w93, "Value"=w92) -> ()  [unwired: 1 in, 2 out]
            n118 = call-poly <vilib>:"DAQmx Write.vi"("task/channels in"=w100, "auto start"=TRUE, "data"=w95, "error in"=w99) -> ("task out"=w101:refnum<k21>, "error out"=w98:errorcluster)  [unwired: 9 in, 1 out]
          }
        }
        n119 = local read "Stop! Local"() -> (w80:bool)
      }
      n120 = Initialize Array(FALSE ("element"), 6 ("dimension size")) -> (w24:bool[])
      n121 = call-poly <vilib>:"DAQmx Write.vi"("task/channels in"=w23, "data"=w24, "error in"=w22) -> ("task out"=w27:refnum<k21>, "error out"=w26:errorcluster)  [unwired: 10 in, 1 out]
      n122 = call <vilib>:"DAQmx Clear Task.vi"("task in"=w27, "error in"=w26) -> ("error out"=w42:errorcluster)  [unwired: 13 in]
      n123 = call <vilib>:"Simple Error Handler.vi"("type of dialog (OK msg:1)"=w40, "error in (no error)"=w42) -> ()  [unwired: 3 in, 5 out]
    }
    frame #2 {
      n124 = Unbundle By Name(w371) -> ("Heaters"=w370:refnum<vi>)
      n125 = call "Display Message to User"("Enable"=FALSE) -> ("OK"=→"Stopped!":bool)  [unwired: 9 in, 1 out]
      n126 = property class="Bool (strict)"(reference=w370, "Value"=FALSE) -> ()  [unwired: 1 in, 2 out]
    }
  }
  n127 = register-events("Stop! Refnum") -> (reference out=w3:refnum<event-registration>)  [unwired: 2 in, 1 out]
  n128 = while {
    tunnel: w3 -> [w377]
    shift-right: [-1] -> _
    shift-left: 0 -> [w376]
    stop <- w374 stop-if-true
    n129 = event shown="[1] <Stop! Refnum>: Value Change" {
      selector: w377 -> [_ _]
      dyn-events: _ -> [_ _]
      timeout: w376 -> [_ _]
      tunnel: [FALSE ("Value (Signaling)") w379] -> w374
      event Timeout {
        n130 = event-data() -> ()  [unwired: 1 in, 3 out]
      }
      event Value Change {
        n131 = event-data() -> ("NewVal"=w380:bool)  [unwired: 1 in, 5 out]
        n132 = case shown="True" w380 {
          tunnel: [FALSE ("Value (Signaling)") w383] -> w379
          frame False {
          }
          frame True {
            w383 = TRUE ("Value (Signaling)")
            n133 = control-ref of="Stop! Local"() -> (w382:refnum<vi>)
            n134 = property class="Bool (strict)"(reference=w382, "Val(Sgnl)"=w383) -> ()  [unwired: 1 in, 2 out]
          }
        }
      }
    }
  }
